vi "ResolveLogger.vi"(8 "error in (no error)":errorcluster, 11 "Logger in":refnum<class "Logger.lvclass">) -> (0 "error out":errorcluster, 3 "Logger out":refnum<class "Logger.lvclass">)   [LabVIEW 2026, in "Lumberjack.lvlib" / "Logger.lvclass"]
doc: "Resolves which logger instance a call should use.\nReturns the wired Logger in when it holds a valid manager enqueuer; otherwise falls back to the process-default logger set by Initialize (GetProcessDefault). Returns no instance when neither is available, which the log VIs treat as a no-op passthrough. Pure resolution; sends no messages.\nLumberjack.lvlib, Logger.lvclass, public."
uses:
  Logger.lvclass
  Logger.lvclass/Logger.ctl
  <vilib>/ActorFramework/Message Enqueuer/Message Enqueuer.lvclass
  Lumberjack.lvlib
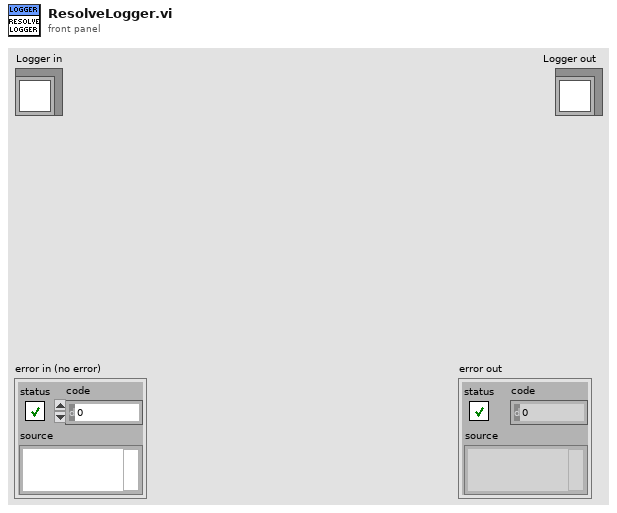
[diagram p1: front panel]
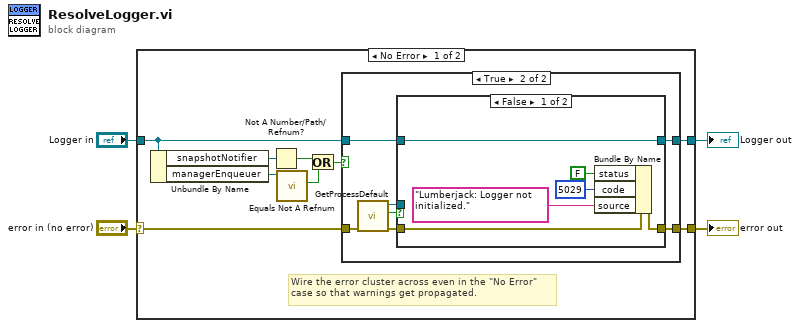
[diagram p0: block diagram]
diagram:
  n1 = case shown="No Error" "error in (no error)" {
    selector: "error in (no error)" -> [w8 w32]
    tunnel: [w6 w32] -> w3
    tunnel: [w7 w31] -> w1
    tunnel: "Logger in" -> [w9 w31]
    frame No Error {
      # "Wire the error cluster across even in the \"No Error\"\ncase so that warnings get propagated."
      n2 = Unbundle By Name(w9) -> ("snapshotNotifier"=w12:refnum<notifier>, "managerEnqueuer"=w13:refnum<class "Message Enqueuer.lvclass">)
      n3 = Not A Number/Path/Refnum?(number/path/refnum=w12) -> (NaN/Path/Refnum?=w11:bool)
      n4 = call <vilib>:"Equals Not A Refnum.vi"("Message Enqueuer"=w13) -> ("Not a refnum?"=w10:bool)  [unwired: 10 in]
      n5 = Or(x=w11, y=w10) -> (x .or. y?=w5:bool)
      n6 = case shown="True" w5 {
        tunnel: w9 -> [w15 w20]
        tunnel: w8 -> [w14 w22]
        tunnel: [w15 w19] -> w7
        tunnel: [w14 w18] -> w6
        frame False {
        }
        frame True {
          n7 = call "GetProcessDefault.vi"("error in (no error)"=w22) -> ("error out"=w21:errorcluster, "found"=w17:bool, "Logger in"=w16:refnum<class "Logger.lvclass">)  [unwired: 8 in]
          n8 = case shown="False" w17 {
            tunnel: w21 -> [w24 w30]
            tunnel: w20 -> [w23 _]
            tunnel: [w23 w29] -> w19
            tunnel: [w26 w30] -> w18
            tunnel: w16 -> [_ w29]
            frame False {
              n9 = Bundle By Name(cluster=w24, "status"=FALSE, "code"=5029, "source"="Lumberjack: Logger not initialized.") -> (w26:errorcluster)
            }
            frame True {
            }
          }
        }
      }
    }
    frame Error {
    }
  }
  "error out" <- w3
  "Logger out" <- w1
